vi "Check_with_Jump.vi"(0 "Current position":sgl[](array[numeric])=[0.0, 200.0, 40.0] format="%.2f", 1 "Traverse Name":string, 3 "Simulate/Run":T1=enum."Run VI", 5 "New Position":sgl[](array[numeric])=[0.0, 100.0, 40.0] format="%.2f", 14 "Model       Roll      Pitch       Yaw (deg)":sgl[](array[numeric]) format="%#.2f") -> (4 "Error Comments":string, 10 "Steps":sgl[][](array[numeric])=[[0.0, 200.0, 40.0]] format="%.2f")   [LabVIEW 2020]
uses:
  Controls/User_Specific_mode.ctl
  Route_mapping_global.vi
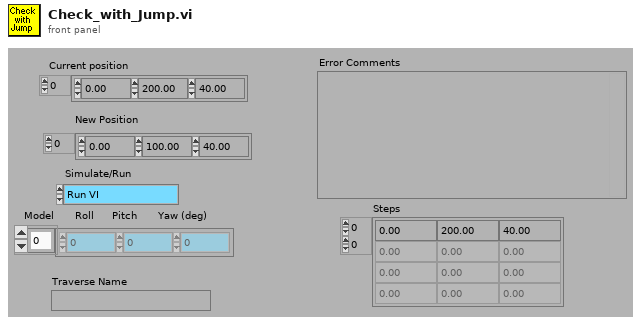
[diagram p1: front panel]
types:
  T1 = typedef "User_Specific_mode.ctl" = enum16{"Check VI only", "Run VI"}
  T2 = typedef "Box_size.ctl" = cluster{"Max":sgl, "Min":sgl}[]
  T3 = typedef "Exclude_cluster.ctl" = cluster{"Sizes":T2, "Name":string, "Exclude Type":T4}
  T4 = typedef "Exclusion_type.ctl" = enum16{"Exclude completely", "Allow only vertical moves"}
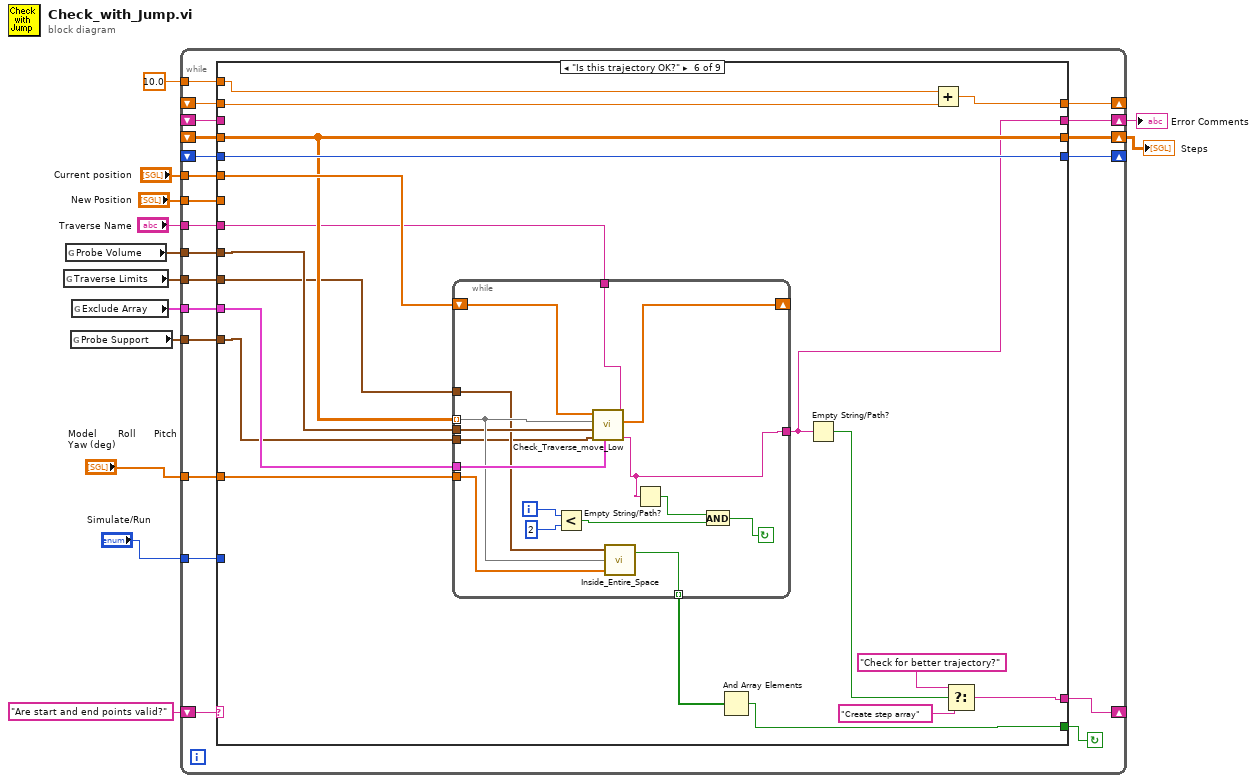
[diagram p0: block diagram]
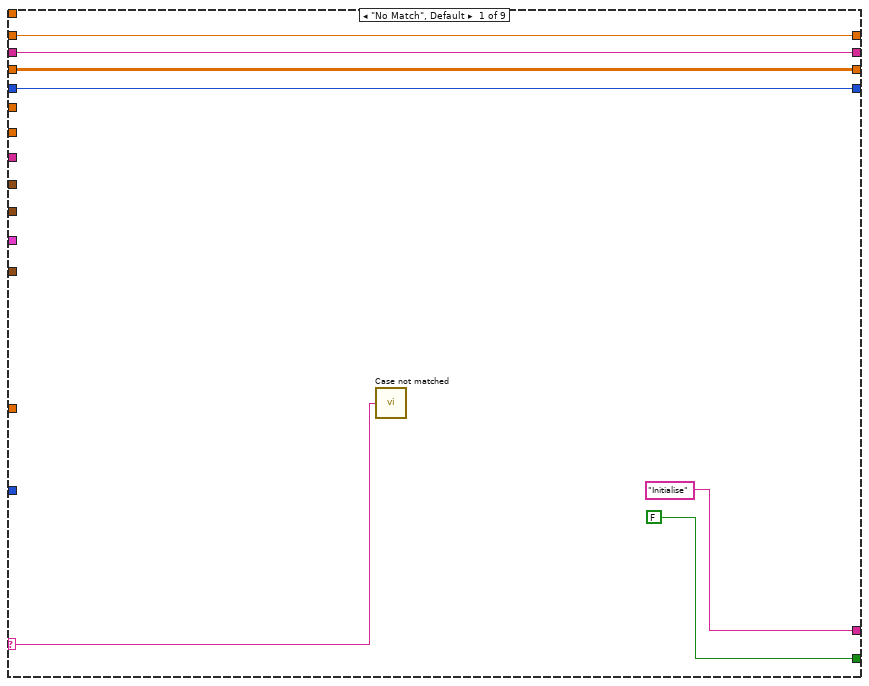
[diagram p2: hidden frame]
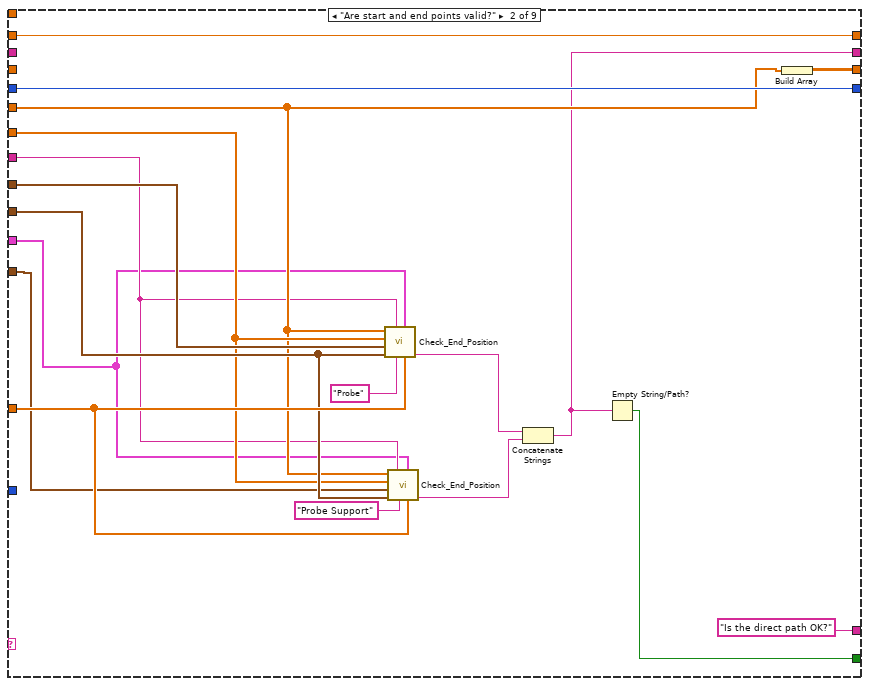
[diagram p3: hidden frame]
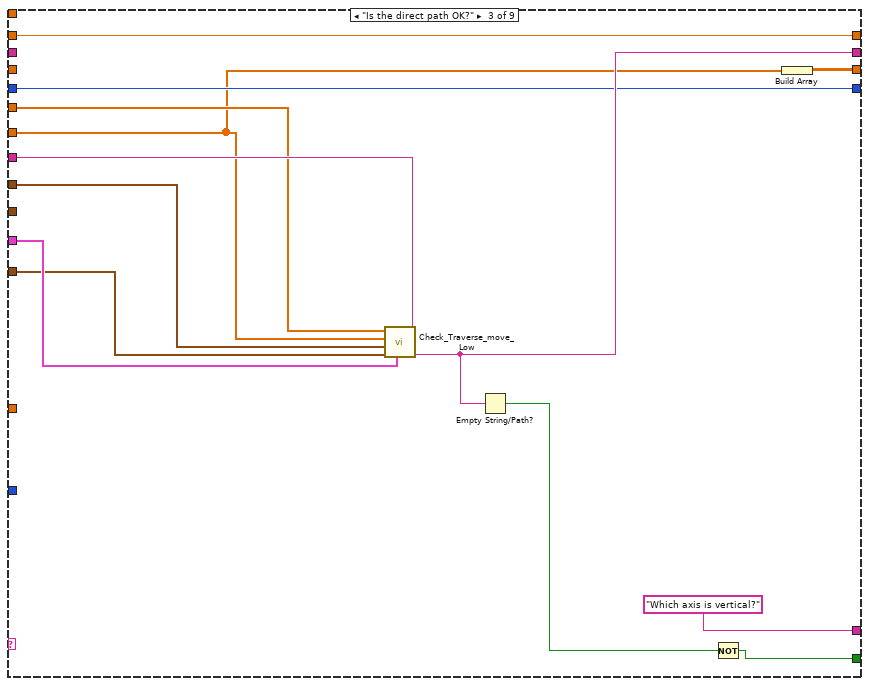
[diagram p4: hidden frame]
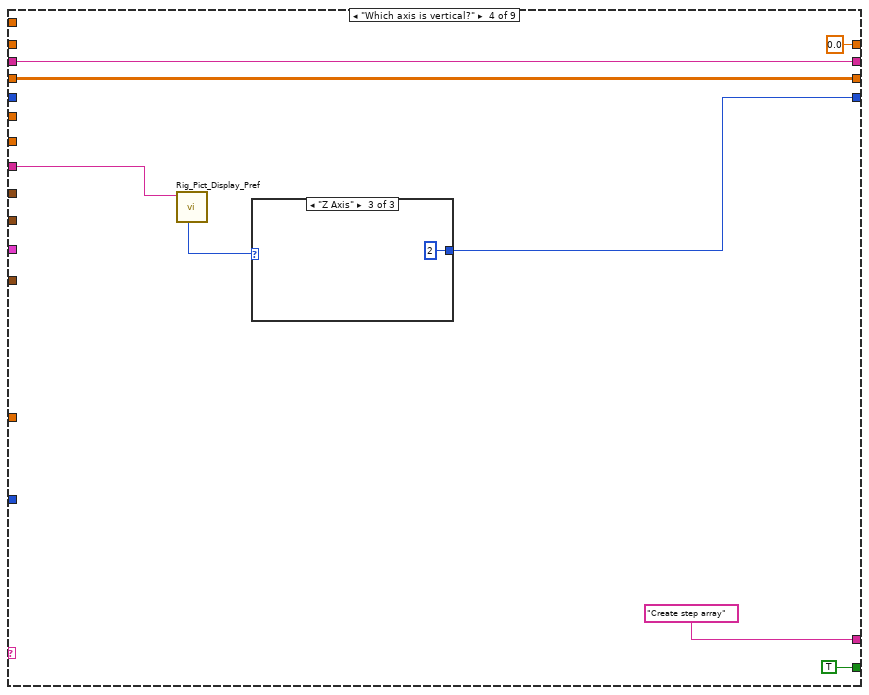
[diagram p5: hidden frame]
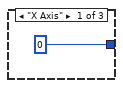
[diagram p6: hidden frame]
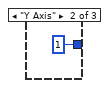
[diagram p7: hidden frame]
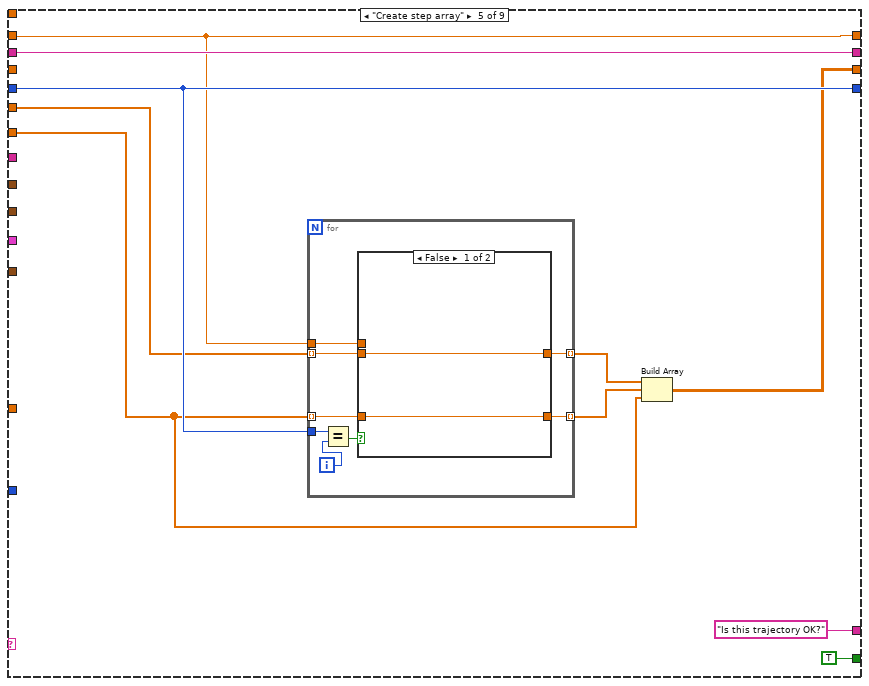
[diagram p8: hidden frame]
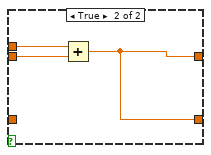
[diagram p9: hidden frame]
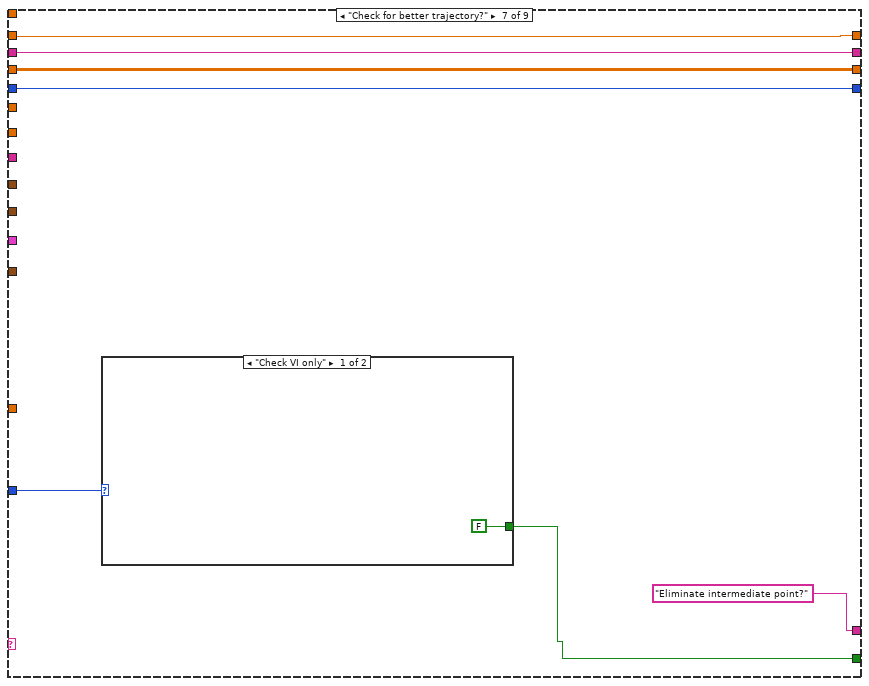
[diagram p10: hidden frame]
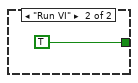
[diagram p11: hidden frame]
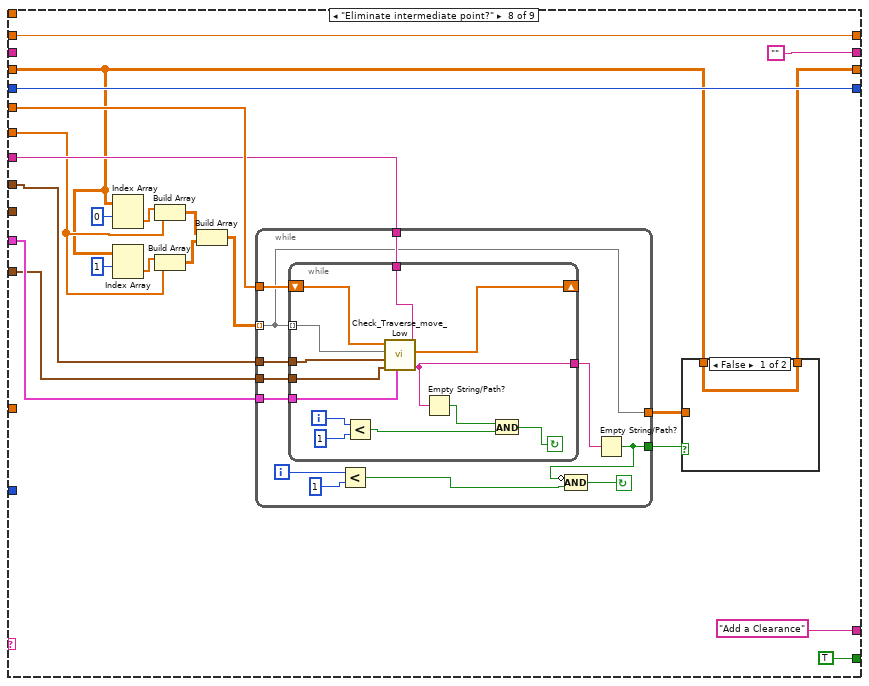
[diagram p12: hidden frame]
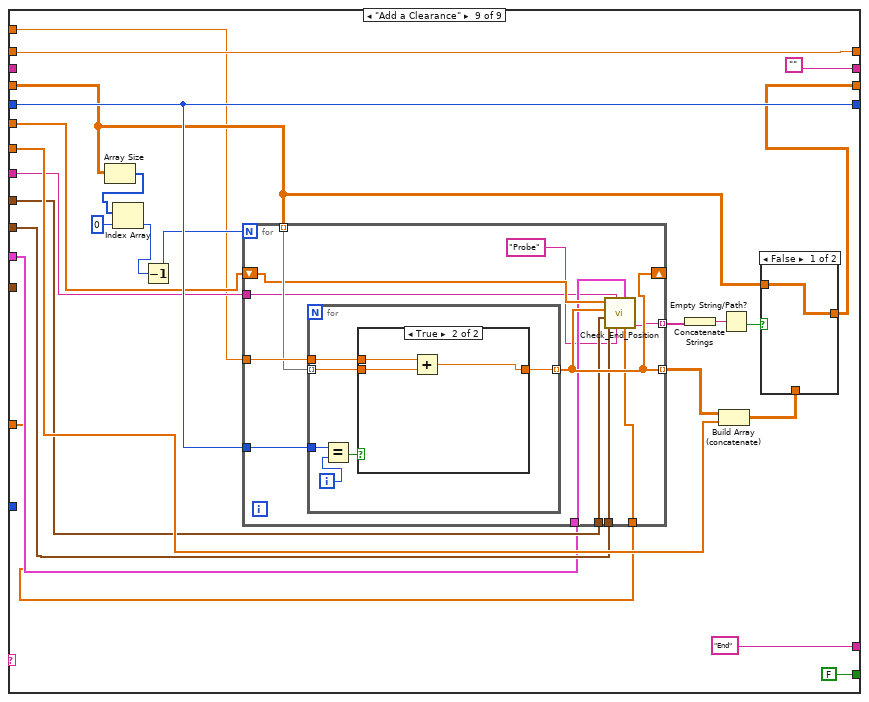
[diagram p14: hidden frame]
diagram:
  n1 = global read "Route_mapping_global.vi" "Traverse Limits"() -> (w2:T2)
  n2 = global read "Route_mapping_global.vi" "Probe Volume"() -> (w1:T2)
  n3 = global read "Route_mapping_global.vi" "Probe Support"() -> (w3:T2)
  n4 = global read "Route_mapping_global.vi" "Exclude Array"() -> (w4:T3[])
  n5 = while {
    shift-left: "Are start and end points valid?" -> [w33]
    shift-right: [w34] -> _
    shift-right: [w30] -> w8
    shift-left: _ -> [w31]
    shift-right: [w29] -> w9
    shift-left: _ -> [w28]
    tunnel: "Current position" -> [w27]
    tunnel: "New Position" -> [w26]
    tunnel: w1 -> [w25]
    tunnel: w2 -> [w24]
    tunnel: w4 -> [w23]
    tunnel: "Traverse Name" -> [w22]
    shift-right: [w21] -> _
    shift-left: _ -> [w20]
    shift-right: [w19] -> _
    shift-left: _ -> [w18]
    tunnel: 10.0 -> [w17]
    tunnel: "Simulate/Run" -> [w16]
    tunnel: "Model       Roll      Pitch       Yaw (deg)" -> [w15]
    tunnel: w3 -> [w14]
    stop <- w32 continue-if-true
    n6 = case shown="\"Is this trajectory OK?\"" w33 {
      selector: w33 -> [w35 _ _ _ _ _ _ _ _]
      tunnel: [FALSE w56 w64 TRUE TRUE w108 w142 TRUE FALSE] -> w32
      tunnel: ["Initialise" "Is the direct path OK?" "Which axis is vertical?" "Create step array" "Is this trajectory OK?" w118 "Eliminate intermediate point?" "Add a Clearance" "End"] -> w34
      tunnel: w31 -> [w39 _ _ w78 w92 _ w148 _ _]
      tunnel: [w39 w45 w68 w78 w92 w115 w148 "" ""] -> w30
      tunnel: [w38 w57 w66 w79 w85 w123 w145 w158 w208] -> w29
      tunnel: w28 -> [w38 _ _ w79 _ w123 w145 w156 w207]
      tunnel: w27 -> [_ w49 w67 _ w89 w124 _ w171 w213]
      tunnel: w26 -> [_ w50 w61 _ w86 _ _ w163 w214]
      tunnel: w25 -> [_ w58 w71 _ _ w122 _ w170 w206]
      tunnel: w24 -> [_ w52 _ _ _ w110 _ _ w205]
      tunnel: w23 -> [_ w42 w70 _ _ w121 _ w169 w204]
      tunnel: w22 -> [_ w48 w69 w77 _ w120 _ w168 w203]
      tunnel: [w37 w55 w63 w75 w90 w125 w147 w172 w221] -> w21
      tunnel: w20 -> [w37 w55 w63 _ w90 w125 w147 w172 w221]
      tunnel: [w36 w54 w62 0.0 w84 w112 w146 w155 w219] -> w19
      tunnel: w18 -> [w36 w54 w62 _ w84 w114 w146 w155 w219]
      tunnel: w17 -> [_ _ _ _ _ w113 _ _ w201]
      tunnel: w16 -> [_ _ _ _ _ _ w144 _ _]
      tunnel: w15 -> [_ w53 _ _ _ w111 _ _ w200]
      tunnel: w14 -> [_ w51 w60 _ _ w107 _ w151 _]
      frame "No Match", Default {
        n7 = call "Case not matched.vi"("Case Name not Matched"=w35) -> ()
      }
      frame "Are start and end points valid?" {
        n8 = call "Check_End_Position.vi"("Model       Roll      Pitch       Yaw (deg)"=w53, "Exclude Array"=w42, "Volume Name"="Probe", "Traverse Name"=w48, "Entire Space"=w52, "Probe Volume"=w58, "New Position"=w50, "Current position"=w49) -> ("Error Comments"=w44:string)  [unwired: 3 in]
        n9 = call "Check_End_Position.vi"("Model       Roll      Pitch       Yaw (deg)"=w53, "Exclude Array"=w42, "Volume Name"="Probe Support", "Traverse Name"=w48, "Entire Space"=w52, "Probe Volume"=w51, "New Position"=w50, "Current position"=w49) -> ("Error Comments"=w43:string)  [unwired: 3 in]
        n10 = Concatenate Strings(w44, w43) -> (w45:string)
        n11 = Empty String/Path?(string/path=w45) -> (empty?=w56:bool)
        n12 = Build Array(w49) -> (w57:sgl[][])
      }
      frame "Is the direct path OK?" {
        n13 = call "Check_Traverse_move_Low.vi"("Traverse Name"=w69, "Exclude Array"=w70, "Probe Support"=w60, "Probe Volume"=w71, "New Position"=w61, "Current position"=w67) -> ("Error Comments"=w68:string)  [unwired: 1 in, 2 out]
        n14 = Empty String/Path?(string/path=w68) -> (empty?=w65:bool)
        n15 = Not(x=w65) -> (.not. x?=w64:bool)
        n16 = Build Array(w61) -> (w66:sgl[][])
      }
      frame "Which axis is vertical?" {
        n17 = call "Rig_Pict_Display_Pref.vi"("Traverse Name"=w77) -> ("Which Axis is vertical?"=w76:enum16{"X Axis", "Y Axis", "Z Axis"})  [unwired: 7 out]
        n18 = case shown="\"Z Axis\"" w76 {
          tunnel: [0 1 2] -> w75
          frame "X Axis" {
          }
          frame "Y Axis" {
          }
          frame "Z Axis" {
          }
        }
      }
      frame "Create step array" {
        n19 = for {
          tunnel: w84 -> [w101]
          tunnel: w90 -> [w98]
          tunnel: w89 -> [w97] mode=indexing
          tunnel: [w96] -> w88 mode=indexing
          tunnel: w86 -> [w95] mode=indexing
          tunnel: [w94] -> w87 mode=indexing
          i -> [w100]
          n20 = Equal?(x=w98, y=w100) -> (x = y?=w99:bool)
          n21 = case shown="False" w99 {
            tunnel: w101 -> [_ w106]
            tunnel: w97 -> [w103 w105]
            tunnel: [w103 w104] -> w96
            tunnel: w95 -> [w102 _]
            tunnel: [w102 w104] -> w94
            frame False {
            }
            frame True {
              n22 = Add(x=w106, y=w105) -> (x+y=w104:dbl)
            }
          }
        }
        n23 = Build Array(w88, w87, w86) -> (w85:dbl[][])
      }
      frame "Is this trajectory OK?" {
        n24 = while {
          shift-right: [w135] -> _
          shift-left: w124 -> [w136]
          tunnel: w123 -> [w132] mode=indexing
          tunnel: w122 -> [w131]
          tunnel: w121 -> [w134]
          tunnel: w120 -> [w126]
          tunnel: [w133] -> w115
          tunnel: w111 -> [w130]
          tunnel: w110 -> [w128]
          tunnel: [w129] -> w109 mode=indexing
          tunnel: w107 -> [w127]
          i -> [w137]
          stop <- w138 continue-if-true
          n25 = Less?(x=w137, y=2 ("x")) -> (x < y?=w139:bool)
          n26 = call "Check_Traverse_move_Low.vi"("Traverse Name"=w126, "Exclude Array"=w134, "Probe Support"=w127, "Probe Volume"=w131, "New Position"=w132, "Current position"=w136) -> ("Error Comments"=w133:string, "Position At Crash"=w135:dbl[])  [unwired: 1 in, 1 out]
          n27 = call "Inside_Entire_Space.vi"("Model       Roll      Pitch       Yaw (deg)"=w130, "Current Position"=w132, "Envelope"=w128) -> ("Box Inside"=w129:bool)  [unwired: 1 in, 1 out]
          n28 = Empty String/Path?(string/path=w133) -> (empty?=w140:bool)
          n29 = And(x=w140, y=w139) -> (x .and. y?=w138:bool)
        }
        n30 = And Array Elements(Boolean array=w109) -> (logical AND=w108:bool)
        n31 = Empty String/Path?(string/path=w115) -> (empty?=w119:bool)
        n32 = Add(x=w113, y=w114) -> (x+y=w112:dbl)
        n33 = Select(t="Check for better trajectory?", s=w119, f="Create step array") -> (s? t:f=w118:string)
      }
      frame "Check for better trajectory?" {
        n34 = case shown="\"Check VI only\"" w144 {
          tunnel: [FALSE TRUE] -> w142
          frame "Check VI only" {
          }
          frame "Run VI" {
          }
        }
      }
      frame "Eliminate intermediate point?" {
        n35 = Index Array(array=w156, index (row)=0) -> (element=w165:dbl[])  [unwired: 1 in]
        n36 = Index Array(array=w156, index (row)=1) -> (element=w164:dbl[])  [unwired: 1 in]
        n37 = Build Array(w165, w163) -> (w162:dbl[][])
        n38 = Build Array(w164, w163) -> (w161:dbl[][])
        n39 = Build Array(w162, w161) -> (w160:dbl[][][])
        n40 = while {
          tunnel: w171 -> [w186]
          tunnel: w170 -> [w185]
          tunnel: w169 -> [w184]
          tunnel: w168 -> [w183]
          tunnel: w160 -> [w176] mode=indexing
          tunnel: [w177] -> w159
          tunnel: [w176] -> w157
          tunnel: w151 -> [w175]
          i -> [w180]
          stop <- w178 continue-if-true
          n41 = while {
            shift-right: [w195] -> _
            shift-left: w186 -> [w199]
            tunnel: w185 -> [w198]
            tunnel: w184 -> [w197]
            tunnel: w183 -> [w196]
            tunnel: [w189] -> w182
            tunnel: w176 -> [w188] mode=indexing
            tunnel: w175 -> [w187]
            i -> [w194]
            stop <- w190 continue-if-true
            n42 = Less?(x=w194, y=1 ("x")) -> (x < y?=w191:bool)
            n43 = call "Check_Traverse_move_Low.vi"("Traverse Name"=w196, "Exclude Array"=w197, "Probe Support"=w187, "Probe Volume"=w198, "New Position"=w188, "Current position"=w199) -> ("Error Comments"=w189:string, "Position At Crash"=w195:dbl[])  [unwired: 1 in, 1 out]
            n44 = Empty String/Path?(string/path=w189) -> (empty?=w192:bool)
            n45 = And(x=w192, y=w191) -> (x .and. y?=w190:bool)
          }
          n46 = Less?(x=w180, y=1 ("x")) -> (x < y?=w179:bool)
          n47 = Empty String/Path?(string/path=w182) -> (empty?=w177:bool)
          n48 = Compound Arithmetic op=AND(invert w177, w179) -> (w178:bool)
        }
        n49 = case shown="False" w159 {
          tunnel: [w173 w174] -> w158
          tunnel: w157 -> [_ w174]
          tunnel: w156 -> [w173 _]
          frame False {
          }
          frame True {
          }
        }
      }
      frame "Add a Clearance" {
        n50 = Array Size(array=w207) -> (size(s)=w218:i32[])
        n51 = Index Array(array=w218, index=0) -> (element=w216:i32)
        n52 = Decrement(x=w216) -> (x-1=w215:i32)
        n53 = for {
          N: w215 -> [_]
          tunnel: w221 -> [w237]
          tunnel: [w233] -> w220 mode=indexing
          tunnel: w201 -> [w236]
          tunnel: w207 -> [w235] mode=indexing
          shift-right: [w233] -> _
          shift-left: w213 -> [w234]
          tunnel: [w232] -> w212 mode=indexing
          tunnel: w206 -> [w231]
          tunnel: w205 -> [w230]
          tunnel: w204 -> [w229]
          tunnel: w203 -> [w228]
          tunnel: w200 -> [w227]
          n54 = for {
            tunnel: w236 -> [w243]
            tunnel: w237 -> [w240]
            tunnel: w235 -> [w239] mode=indexing
            tunnel: [w238] -> w233 mode=indexing
            i -> [w242]
            n55 = Equal?(x=w240, y=w242) -> (x = y?=w241:bool)
            n56 = case shown="True" w241 {
              tunnel: w243 -> [_ w247]
              tunnel: w239 -> [w244 w246]
              tunnel: [w244 w245] -> w238
              frame False {
              }
              frame True {
                n57 = Add(x=w247, y=w246) -> (x+y=w245:dbl)
              }
            }
          }
          n58 = call "Check_End_Position.vi"("Model       Roll      Pitch       Yaw (deg)"=w227, "Exclude Array"=w229, "Volume Name"="Probe", "Traverse Name"=w228, "Entire Space"=w230, "Probe Volume"=w231, "New Position"=w233, "Current position"=w234) -> ("Error Comments"=w232:string)  [unwired: 3 in]
        }
        n59 = Concatenate Strings(w212) -> (w211:string)
        n60 = Build Array (concatenate)(w220, w214) -> (w209:dbl[][])
        n61 = Empty String/Path?(string/path=w211) -> (empty?=w210:bool)
        n62 = case shown="False" w210 {
          tunnel: w209 -> [_ w225]
          tunnel: [w224 w225] -> w208
          tunnel: w207 -> [w224 _]
          frame False {
          }
          frame True {
          }
        }
      }
    }
  }
  "Error Comments" <- w8
  "Steps" <- w9
